vi "Set All Controls Status.vi"(8 "String":string, 10 "UI Refs":T8, 11 "Config":T1 {"Hardware Configuration"."Lasers Configuration"."SettingValues"."785 Power" format="%.1f"; "Hardware Configuration"."Lasers Configuration"."SettingValues"."647 Power" format="%.1f"; "Hardware Configuration"."Lasers Configuration"."SettingValues"."561 Power" format="%.1f"; "Hardware Configuration"."Lasers Configuration"."SettingValues"."532 Power" format="%.1f"; "Hardware Configuration"."Lasers Configuration"."SettingValues"."488 Power" format="%.1f"; "Hardware Configuration"."Lasers Configuration"."SettingValues"."405 Power" format="%.1f"}) -> ()   [LabVIEW 2019]
uses:
  controls/UI Data.ctl
  Settings/Settings.ctl
  HardwareAdapter/Support/Hardware Configuration.ctl
  HardwareAdapter/Support/Camera Configuration.ctl
  D:/SDK/PMQI-LabViewSamples/Examples/Dependencies/PVCamNET.dll
  <vilib>/userdefined/High Color/IMAQdx.ctl
  E:/DevHardSoftware/MMicroscopy/HardwareAdapter/Lasers/Dependencies/Oxxius_Boxx.dll
  HardwareAdapter/Lasers/Dependencies/Oxxius_Boxx.dll
  Logging/Logging Configuration.ctl
  controls/UI Configuration.ctl
  controls/CallBack Refs.ctl
  Logging/Logging.lvlib
  Settings/Settings.lvlib
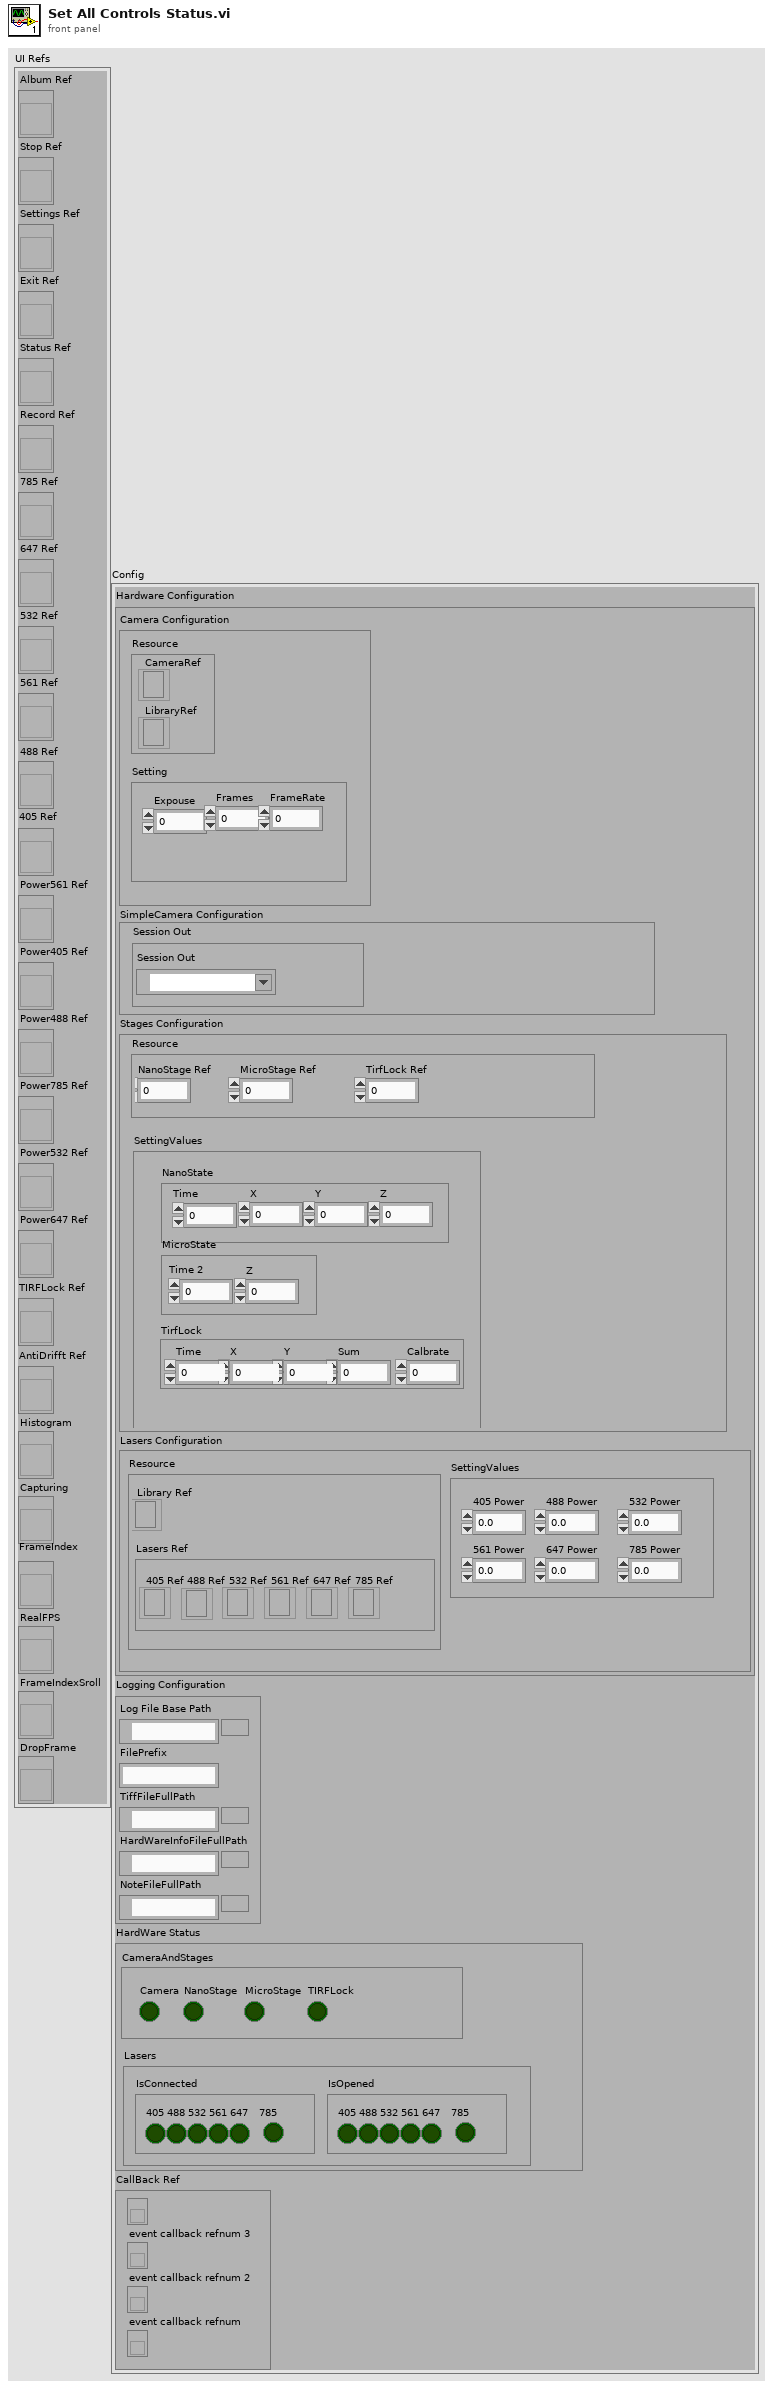
[diagram p1: front panel]
types:
  T1 = typedef "Settings.lvlib/Settings.ctl" = cluster{"Hardware Configuration":T2, "Logging Configuration":T5, "HardWare Status":cluster{"CameraAndStages":T6, "Lasers":cluster{"IsConnected":cluster{"405":bool, "488":bool, "532":bool, "561":bool, "647":bool, "785":bool}, "IsOpened":cluster{"405":bool, "488":bool, "532":bool, "561":bool, "647":bool, "785":bool}}}, "CallBack Ref":T7}
  T2 = typedef "Hardware Configuration.ctl" = cluster{"Camera Configuration":T3, "SimpleCamera Configuration":cluster{"Resource":cluster{"Session Out":T4}}, "Stages Configuration":cluster{"Resource":cluster{"NanoStage Ref":i32, "MicroStage Ref":i32, "TirfLock Ref":i32}, "SettingValues":cluster{"NanoState":cluster{"Time":dbl, "X":dbl, "Y":dbl, "Z":dbl}, "MicroState":cluster{"Time 2":dbl, "Z":dbl}, "TirfLock":cluster{"Time":dbl, "X":dbl, "Y":dbl, "Sum":dbl, "Calbrate":dbl}}}, "Lasers Configuration":cluster{"SettingValues":cluster{"405 Power":sgl, "488 Power":sgl, "532 Power":sgl, "561 Power":sgl, "647 Power":sgl, "785 Power":sgl}, "Resource":cluster{"Library Ref":refnum<k24>, "Lasers Ref":cluster{"405 Ref":refnum<k24>, "488 Ref":refnum<k24>, "532 Ref":refnum<k24>, "561 Ref":refnum<k24>, "647 Ref":refnum<k24>, "785 Ref":refnum<k24>}}}}
  T3 = typedef "Camera Configuration.ctl" = cluster{"Resource":cluster{"CameraRef":refnum<k24>, "LibraryRef":refnum<k24>}, "Setting":cluster{"Expouse":dbl, "Frames":dbl, "FrameRate":dbl}}
  T4 = typedef "IMAQdx.ctl" = refnum<k21>
  T5 = typedef "Logging.lvlib/Logging Configuration.ctl" = cluster{"Log File Base Path":path, "FilePrefix":string, "TiffFileFullPath":path, "HardWareInfoFileFullPath":path, "NoteFileFullPath":path}
  T6 = typedef "UI Configuration.ctl" = cluster{"Camera":bool, "NanoStage":bool, "MicroStage":bool, "TIRFLock":bool}
  T7 = typedef "CallBack Refs.ctl" = cluster{"event callback refnum":refnum<k27>, "event callback refnum 2":refnum<k27>, "event callback refnum 3":refnum<k27>, "event callback refnum 4":refnum<k27>}
  T8 = typedef "UI Data.ctl" = cluster{"Album Ref":refnum<vi>, "Stop Ref":refnum<vi>, "Settings Ref":refnum<vi>, "Exit Ref":refnum<vi>, "Status Ref":refnum<vi>, "Record Ref":refnum<vi>, "785 Ref":refnum<vi>, "647 Ref":refnum<vi>, "532 Ref":refnum<vi>, "561 Ref":refnum<vi>, "488 Ref":refnum<vi>, "405 Ref":refnum<vi>, "Power561 Ref":refnum<vi>, "Power405 Ref":refnum<vi>, "Power488 Ref":refnum<vi>, "Power785 Ref":refnum<vi>, "Power532 Ref":refnum<vi>, "Power647 Ref":refnum<vi>, "TIRFLock Ref":refnum<vi>, "AntiDrifft Ref":refnum<vi>, "Histogram":refnum<vi>, "Capturing":refnum<vi>, "FrameIndex":refnum<vi>, "RealFPS":refnum<vi>, "FrameIndexSroll":refnum<vi>, "DropFrame":refnum<vi>}
  T9 = cluster{"405":bool, "488":bool, "532":bool, "561":bool, "647":bool, "785":bool}
  T10 = cluster{"405 Power":sgl, "488 Power":sgl, "532 Power":sgl, "561 Power":sgl, "647 Power":sgl, "785 Power":sgl}
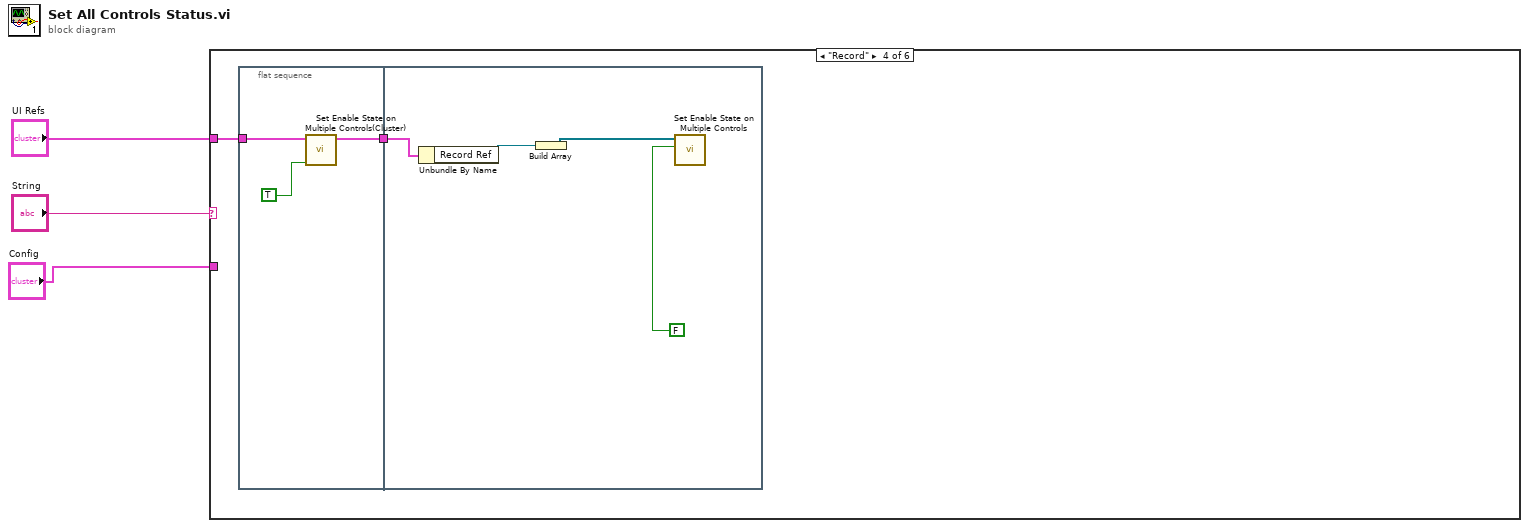
[diagram p0: block diagram]
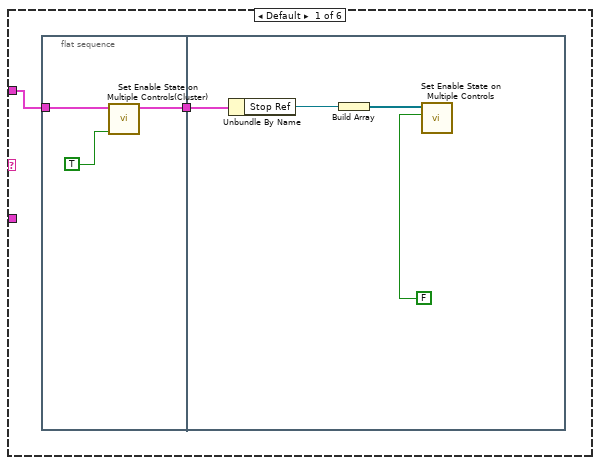
[diagram p2: hidden frame]
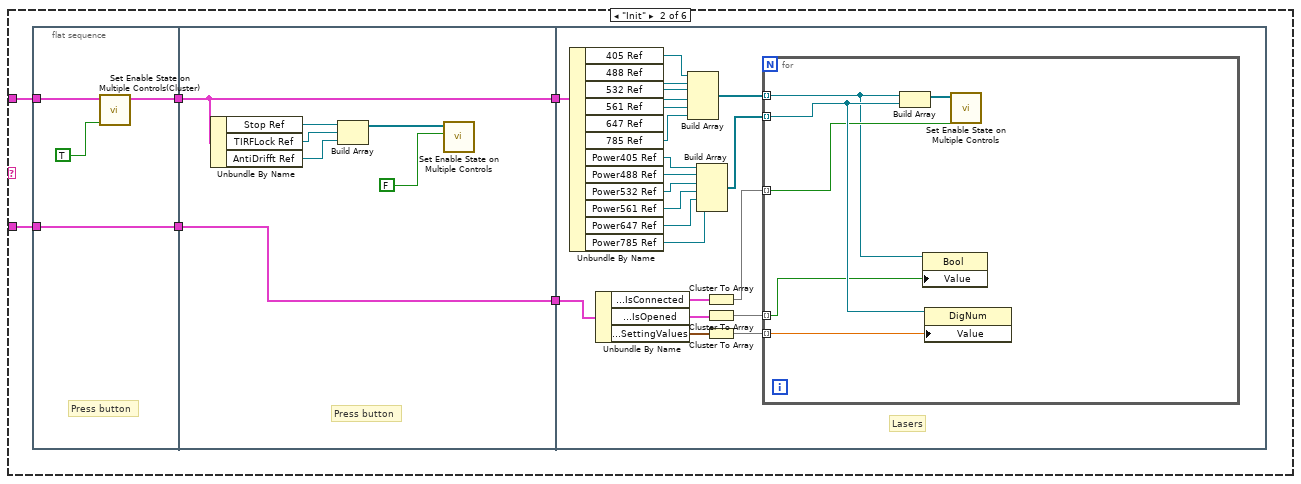
[diagram p3: hidden frame]
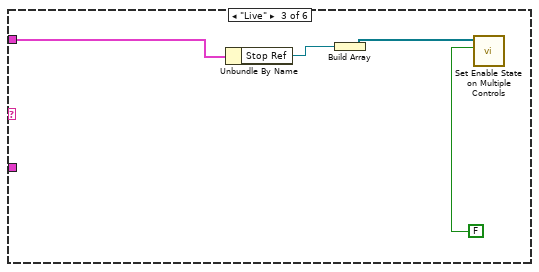
[diagram p4: hidden frame]
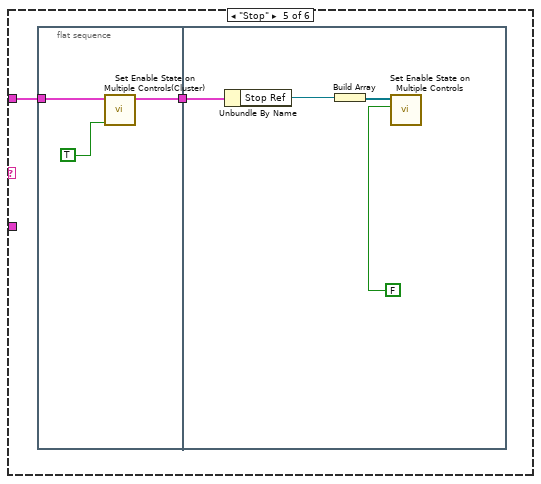
[diagram p5: hidden frame]
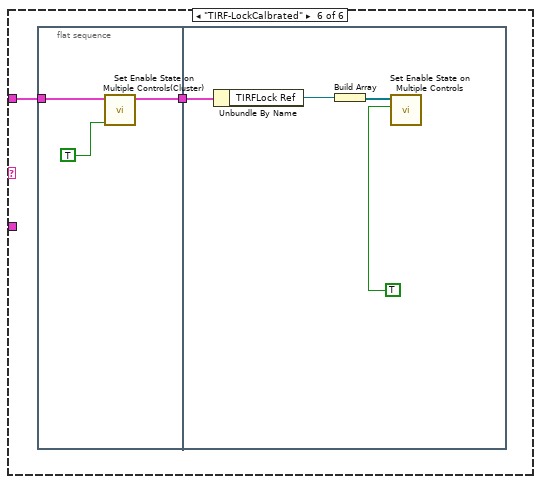
[diagram p6: hidden frame]
diagram:
  n1 = case shown="\"Record\"" "String" {
    tunnel: "UI Refs" -> [w4 w18 w58 w63 w72 w81]
    tunnel: "Config" -> [_ w14 _ _ _ _]
    frame Default {
      n2 = flat-sequence {
        tunnel: w4 -> [w8]
        tunnel: [w6] -> w5
        tunnel: w5 -> [w12]
        frame #0 {
          n3 = call "Set Enable State on Multiple Controls(Cluster).vi"("Enable?"=TRUE, "UI Refs"=w8) -> ("UI Ref Out"=w6:T8)  [unwired: 9 in]
        }
        frame #1 {
          n4 = Unbundle By Name(w12) -> ("Stop Ref"=w11:refnum<vi>)
          n5 = Build Array(w11) -> (w10:refnum<vi>[])
          n6 = call "Set Enable State on Multiple Controls.vi"("Enable?"=FALSE, "Controls"=w10) -> ()  [unwired: 10 in]
        }
      }
    }
    frame "Init" {
      n7 = flat-sequence {
        tunnel: w18 -> [w22]
        tunnel: [w20] -> w17
        tunnel: [w19] -> w15
        tunnel: w14 -> [w19]
        tunnel: w17 -> [w26]
        tunnel: [w26] -> w16
        tunnel: w15 -> [w25]
        tunnel: [w25] -> w13
        tunnel: w16 -> [w51]
        tunnel: w13 -> [w50]
        frame #0 {
          # "Press button"
          n8 = call "Set Enable State on Multiple Controls(Cluster).vi"("Enable?"=TRUE, "UI Refs"=w22) -> ("UI Ref Out"=w20:T8)  [unwired: 9 in]
        }
        frame #1 {
          # "Press button"
          n9 = Unbundle By Name(w26) -> ("Stop Ref"=w29:refnum<vi>, "TIRFLock Ref"=w24:refnum<vi>, "AntiDrifft Ref"=w23:refnum<vi>)
          n10 = Build Array(w29, w24, w23) -> (w28:refnum<vi>[])
          n11 = call "Set Enable State on Multiple Controls.vi"("Enable?"=FALSE, "Controls"=w28) -> ()  [unwired: 10 in]
        }
        frame #2 {
          # "Lasers"
          n12 = Unbundle By Name(w51) -> ("405 Ref"=w47:refnum<vi>, "488 Ref"=w46:refnum<vi>, "532 Ref"=w45:refnum<vi>, "561 Ref"=w44:refnum<vi>, "647 Ref"=w43:refnum<vi>, "785 Ref"=w42:refnum<vi>, "Power405 Ref"=w40:refnum<vi>, "Power488 Ref"=w39:refnum<vi>, "Power532 Ref"=w38:refnum<vi>, "Power561 Ref"=w37:refnum<vi>, "Power647 Ref"=w36:refnum<vi>, "Power785 Ref"=w35:refnum<vi>)
          n13 = Unbundle By Name(w50) -> ("HardWare Status.Lasers.IsConnected"=w49:T9, "HardWare Status.Lasers.IsOpened"=w31:T9, "Hardware Configuration.Lasers Configuration.SettingValues"=w32:T10)
          n14 = Build Array(w47, w46, w45, w44, w43, w42) -> (w41:refnum<vi>[])
          n15 = Build Array(w40, w39, w38, w37, w36, w35) -> (w34:refnum<vi>[])
          n16 = Cluster To Array(cluster=w49) -> (array=w48:bool[])
          n17 = Cluster To Array(cluster=w31) -> (array=w30:bool[])
          n18 = Cluster To Array(cluster=w32) -> (array=w33:sgl[])
          n19 = for {
            tunnel: w48 -> [w55] mode=indexing
            tunnel: w41 -> [w54] mode=indexing
            tunnel: w34 -> [w56] mode=indexing
            tunnel: w33 -> [w53] mode=indexing
            tunnel: w30 -> [w52] mode=indexing
            n20 = Build Array(w54, w56) -> (w57:refnum<vi>[])
            n21 = property class="Bool"(reference=w54, "Value"=w52) -> ()  [unwired: 1 in, 2 out]
            n22 = property class="DigNum"(reference=w56, "Value"=w53) -> ()  [unwired: 1 in, 2 out]
            n23 = call "Set Enable State on Multiple Controls.vi"("Enable?"=w55, "Controls"=w57) -> ()  [unwired: 10 in]
          }
        }
      }
    }
    frame "Live" {
      n24 = Unbundle By Name(w58) -> ("Stop Ref"=w59:refnum<vi>)
      n25 = Build Array(w59) -> (w61:refnum<vi>[])
      n26 = call "Set Enable State on Multiple Controls.vi"("Enable?"=FALSE, "Controls"=w61) -> ()  [unwired: 10 in]
    }
    frame "Record" {
      n27 = flat-sequence {
        tunnel: w63 -> [w66]
        tunnel: [w64] -> w62
        tunnel: w62 -> [w70]
        frame #0 {
          n28 = call "Set Enable State on Multiple Controls(Cluster).vi"("Enable?"=TRUE, "UI Refs"=w66) -> ("UI Ref Out"=w64:T8)  [unwired: 9 in]
        }
        frame #1 {
          n29 = Unbundle By Name(w70) -> ("Record Ref"=w67:refnum<vi>)
          n30 = Build Array(w67) -> (w69:refnum<vi>[])
          n31 = call "Set Enable State on Multiple Controls.vi"("Enable?"=FALSE, "Controls"=w69) -> ()  [unwired: 10 in]
        }
      }
    }
    frame "Stop" {
      n32 = flat-sequence {
        tunnel: w72 -> [w75]
        tunnel: [w73] -> w71
        tunnel: w71 -> [w79]
        frame #0 {
          n33 = call "Set Enable State on Multiple Controls(Cluster).vi"("Enable?"=TRUE, "UI Refs"=w75) -> ("UI Ref Out"=w73:T8)  [unwired: 9 in]
        }
        frame #1 {
          n34 = Unbundle By Name(w79) -> ("Stop Ref"=w78:refnum<vi>)
          n35 = Build Array(w78) -> (w77:refnum<vi>[])
          n36 = call "Set Enable State on Multiple Controls.vi"("Enable?"=FALSE, "Controls"=w77) -> ()  [unwired: 10 in]
        }
      }
    }
    frame "TIRF-LockCalbrated" {
      n37 = flat-sequence {
        tunnel: w81 -> [w84]
        tunnel: [w82] -> w80
        tunnel: w80 -> [w88]
        frame #0 {
          n38 = call "Set Enable State on Multiple Controls(Cluster).vi"("Enable?"=TRUE, "UI Refs"=w84) -> ("UI Ref Out"=w82:T8)  [unwired: 9 in]
        }
        frame #1 {
          n39 = Unbundle By Name(w88) -> ("TIRFLock Ref"=w87:refnum<vi>)
          n40 = Build Array(w87) -> (w86:refnum<vi>[])
          n41 = call "Set Enable State on Multiple Controls.vi"("Enable?"=TRUE, "Controls"=w86) -> ()  [unwired: 10 in]
        }
      }
    }
  }
